vi "Main_ch.vi"() -> ()   [LabVIEW 2020]
uses:
  <vilib>/Utility/error.llb/DialogType.ctl
  <vilib>/DAQmx/read.llb/DAQmx Read (Analog 1D Wfm NChan NSamp).vi
  <extravilib>/ChannelInstances/Tag-bool/Read With Abort.vi
  <extravilib>/ChannelInstances/Tag-bool/Write With Abort.vi
  <vilib>/ULx/Create Channel.llb/ULx Create Channel (AI-Voltage-Basic).vi
  <vilib>/ULx/Timing.llb/ULx Timing (Sample Clock).vi
  <vilib>/DAQmx/create/channels.llb/DAQmx Create Channel (AI-Acceleration-Accelerometer).vi
  <vilib>/DAQmx/configure/timing.llb/DAQmx Timing (Sample Clock).vi
  <vilib>/DAQmx/configure/trigger.llb/DAQmx Start Trigger (Digital Edge).vi
  <vilib>/DAQmx/configure/trigger.llb/DAQmx Start Trigger (Time).vi
  <vilib>/DAQmx/configure/trigger.llb/DAQmx Start Trigger (Analog Edge).vi
  <extravilib>/ChannelInstances/Tag-bool/Instantiate.vi
  <extravilib>/ChannelInstances/Tag-bool/EndpointRead.vi
  <vilib>/ULx/Read.llb/ULx Read (Analog Wfm 1Chan NSamp).vi
  <vilib>/DAQmx/miscellaneous.llb/DAQmx Fill In Error Info.vi
  <vilib>/ULx/Read.llb/ULx Read (Analog 1D Wfm NChan NSamp).vi
  <instrlib>/Tektronix DPO MSO 2000 4000 Series/Public/Data/Read (Multiple Waveforms).vi
  <vilib>/Waveform/WDTFileIO.llb/Export Waveforms To Spreadsheet File (1D).vi
  <extravilib>/ChannelInstances/Tag-bool/Endpoint.vi
  <extravilib>/ChannelInstances/Tag-bool.lvlib
  <instrlib>/Tektronix DPO MSO 2000 4000 Series/Tektronix DPO MSO 2000 4000 Series.lvlib
  <resource>/objmgr/daqmx.rc
panel:
  out "Power Graph":waveform(dbl)[](graph)
  out "Torque Graph":waveform(dbl)(graph)
  in  "Trigger Type":T1(tab)
  in  "Digital Start Trigger Edge":i32(ring)=10280 caption="Edge" items=["Rising"=10280, "Falling"=10171]
  in  "Digital Start Trigger Source":tag="/Dev1/PFI0" caption="Source"
  in  "Digital Pause Trigger Pause When":i32(ring)=10192 caption="Pause When" items=["High"=10192, "Low"=10214]
  in  "Digital Pause Trigger Source":tag="/Dev1/PFI0" caption="Source"
  in  "Analog Start Trigger Level":dbl caption="Level" format="%0.2f"
  in  "Analog Start Trigger Hysteresis":dbl caption="Hysteresis" format="%.2f"
  in  "Analog Start Trigger Slope":i32(ring)=10280 caption="Slope" items=["Rising"=10280, "Falling"=10171]
  in  "Analog Start Trigger Source":string="APFI0" caption="Source"
  in  "Analog Pause Trigger Source":string="APFI0" caption="Source"
  in  "Analog Pause Trigger Pause When":i32(ring)=10093 caption="Pause When" items=["Above Level"=10093, "Below Level"=10107]
  in  "Analog Pause Trigger Level":dbl caption="Level" format="%.2f"
  in  "When":timestamp
  in  "Select Time\nManually":bool
  out "Waveform Graph":waveform(dbl)[](graph)
  out "Actual Sample Rate":dbl=1000.0 format="%0.2f"
  out "Mic Graph":dynamicdata(graph)
  out "Load Cell Graph":waveform(dbl)[](graph)
  in  "stop":bool
  # "To enable triggers, select a tab above, and configure the settings.\n\nNot all hardware supports all trigger types. Refer to your device documentation for more information."
  # "This trigger type is not supported in continuous sample timing. \n\nRefer to your device documentation for more information on which triggers are supported."
  # "This trigger type is not supported in continuous sample timing. \n\nRefer to your device documentation for more information on which triggers are supported."
  # "If time is not manually set, task will begin after 10 seconds"
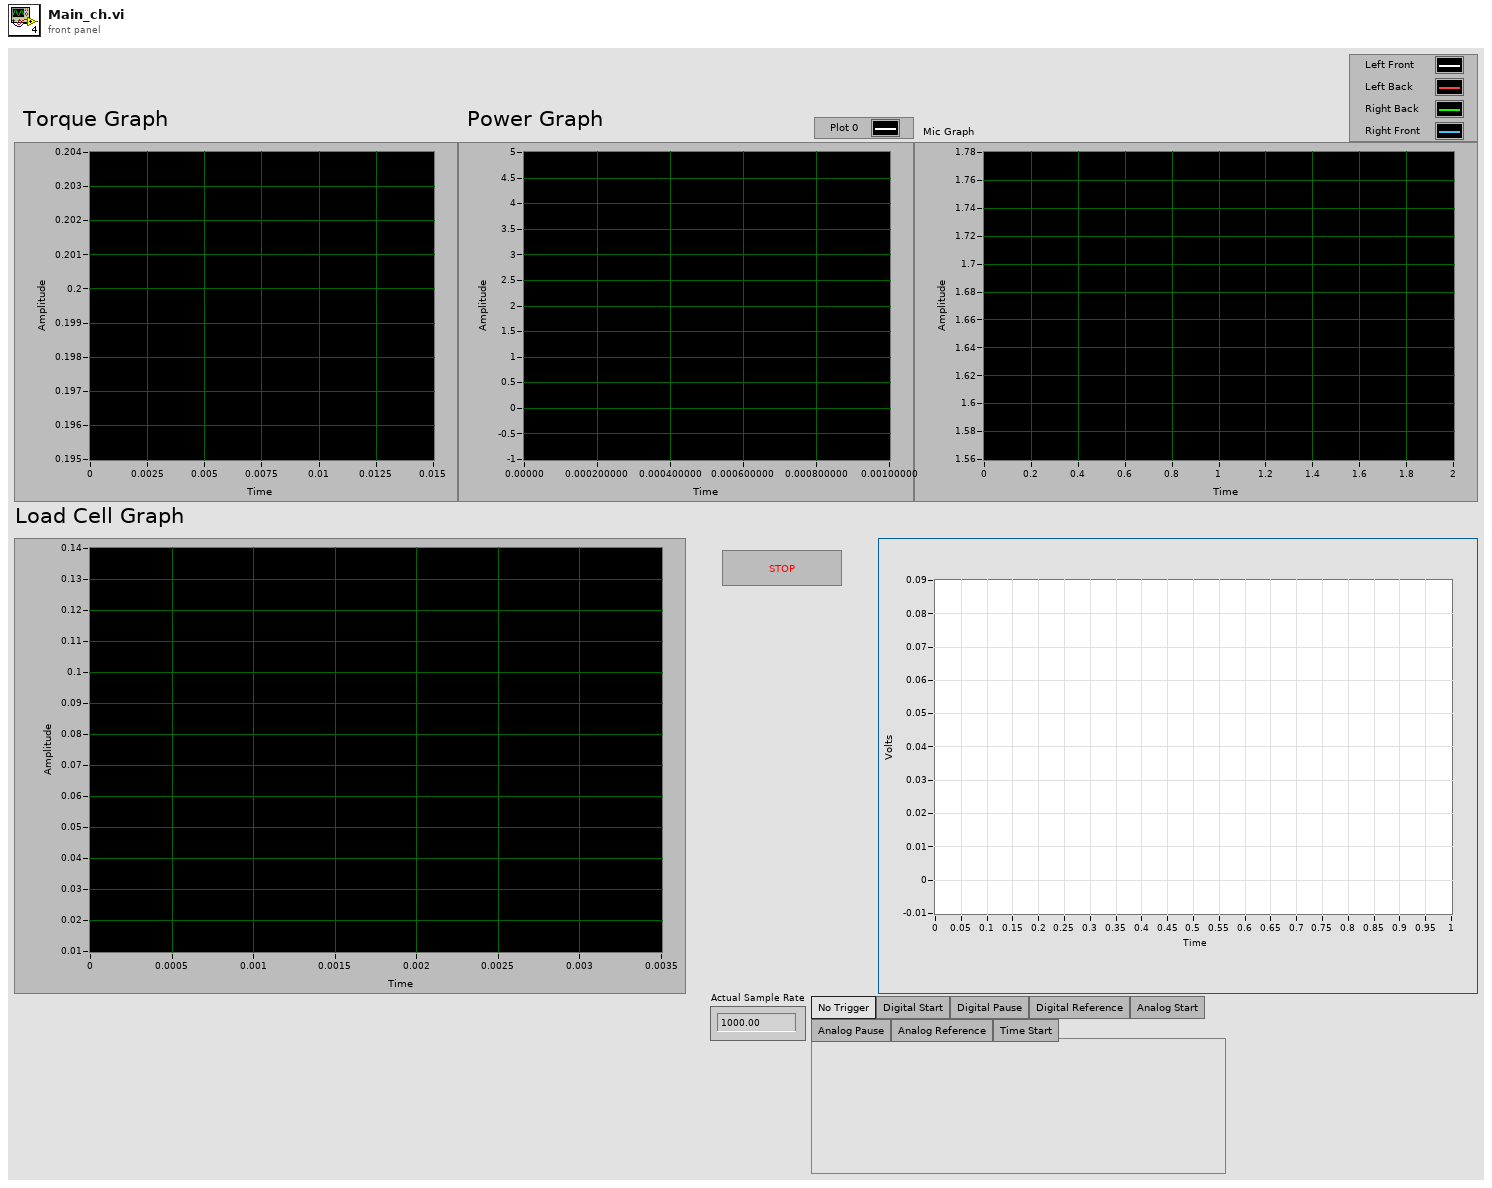
[diagram p1: front panel]
types:
  T1 = enum32{"No Trigger", "Digital Start", "Digital Pause", "Digital Reference", "Analog Start", "Analog Pause", "Analog Reference", "Time Start"}
  T2 = typedef "DialogType.ctl" = u16
  T3 = typedef "Tag-bool.lvlib/))Channel.ctl" = refnum<queue>
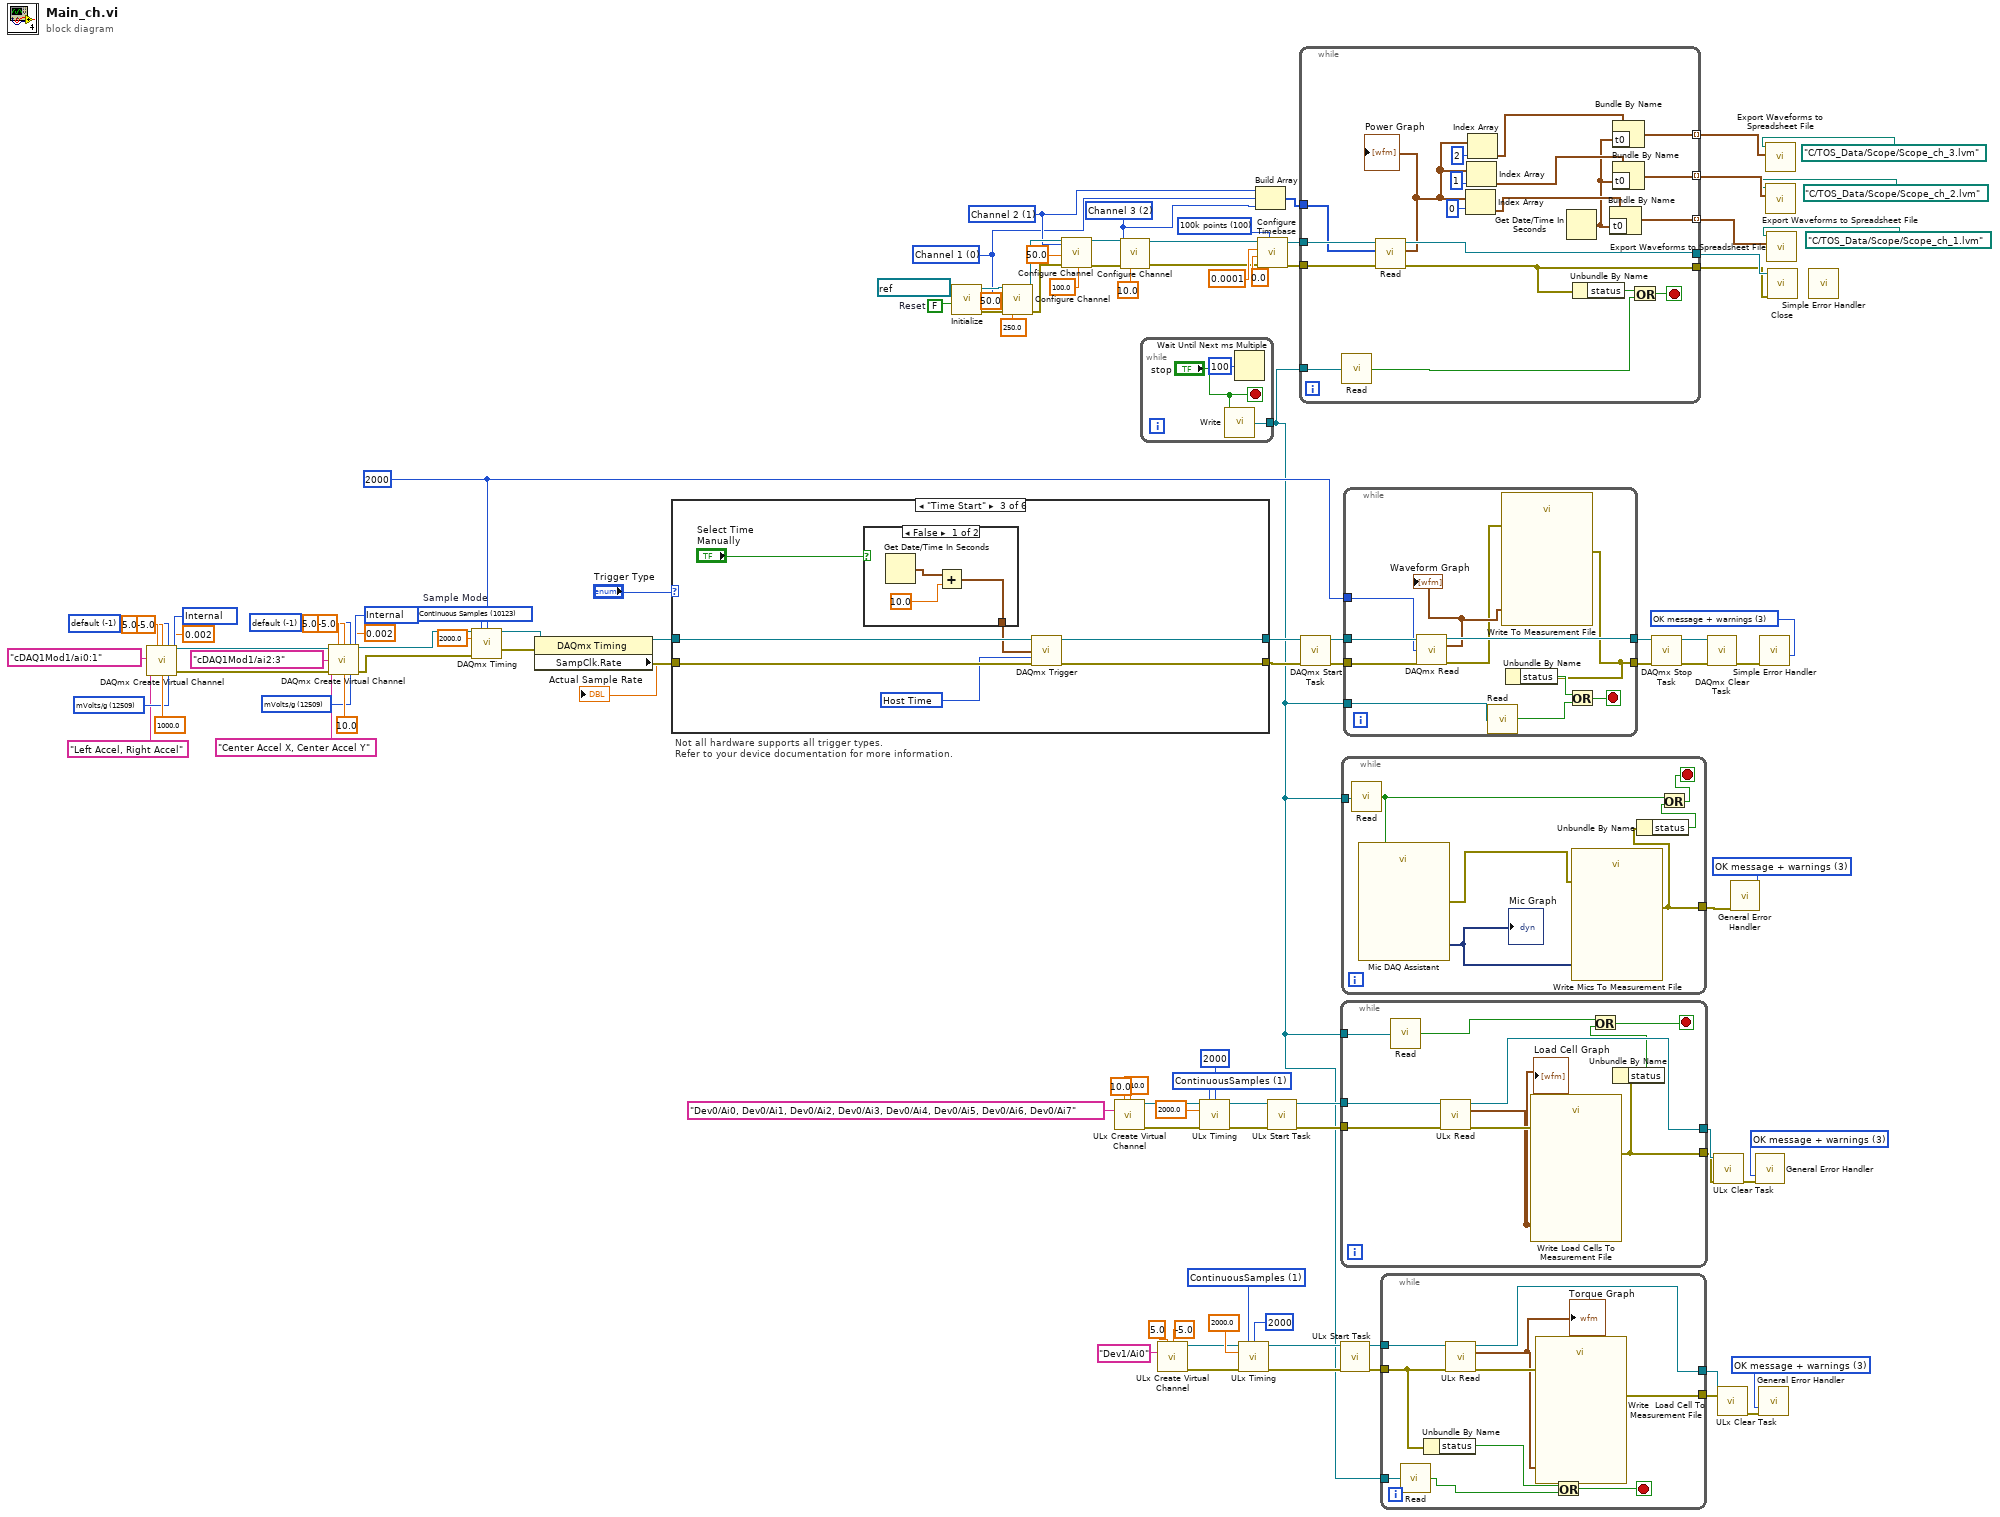
[diagram p0: block diagram]
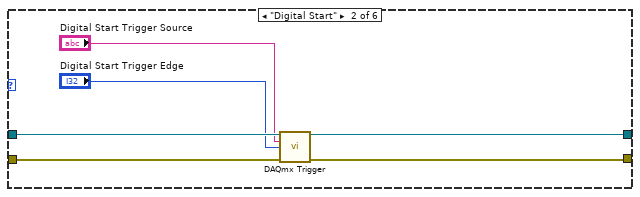
[diagram p3: hidden frame]
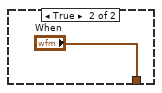
[diagram p4: hidden frame]
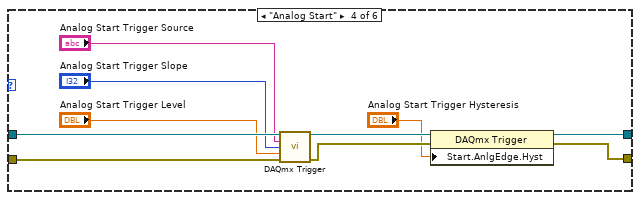
[diagram p5: hidden frame]
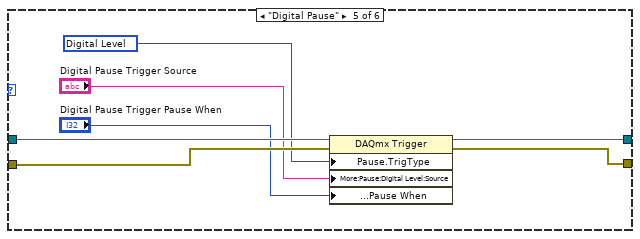
[diagram p6: hidden frame]
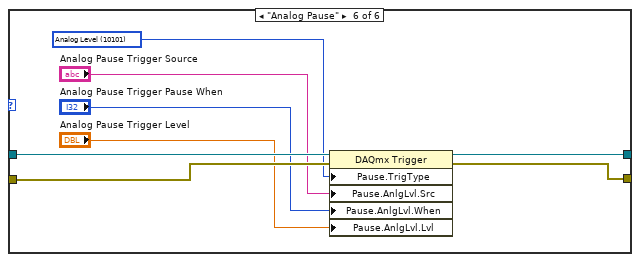
[diagram p7: hidden frame]
diagram:
  w13 = u16 2 items=["Channel 1", "Channel 2", "Channel 3", "Channel 4", "Math", "Reference 1", "Reference 2", "Reference 3", "Reference 4", "Bus 1", "Bus 2"] ("Channel (0: Channel 1)")
  w31 = 1 items=["FiniteSamples", "ContinuousSamples"] ("sample mode")
  w28 = T2 3 items=["no dialog", "OK message", "continue or stop message", "OK message + warnings", "continue/stop + warnings"] ("type of dialog (OK msg:1)")
  w46 = 12509 items=["mVolts/g"=12509, "Volts/g"=12510] ("sensitivity units")
  w47 = 12509 items=["mVolts/g"=12509, "Volts/g"=12510] ("sensitivity units")
  w51 = 10200 items=["Internal"=10200, "External"=10167, "None"=10230] ("current excitation source")
  w52 = -1 items=["default"=-1, "RSE"=10083, "NRSE"=10078, "Differential"=10106, "Pseudodifferential"=12529] ("input terminal configuration")
  w56 = 2000 ("samples per channel")
  w61 = T2 3 items=["no dialog", "OK message", "continue or stop message", "OK message + warnings", "continue/stop + warnings"] ("type of dialog (OK msg:1)")
  w72 = 10123 items=["Finite Samples"=10178, "Continuous Samples"=10123, "Hardware Timed Single Point"=12522]  # Sample Mode
  w76 = 10200 items=["Internal"=10200, "External"=10167, "None"=10230] ("current excitation source")
  w77 = -1 items=["default"=-1, "RSE"=10083, "NRSE"=10078, "Differential"=10106, "Pseudodifferential"=12529] ("input terminal configuration")
  w81 = T2 3 items=["no dialog", "OK message", "continue or stop message", "OK message + warnings", "continue/stop + warnings"] ("type of dialog (OK msg:1)")
  w41 = u16 1 items=["Channel 1", "Channel 2", "Channel 3", "Channel 4", "Math", "Reference 1", "Reference 2", "Reference 3", "Reference 4", "Bus 1", "Bus 2"] ("Channel (0: Channel 1)")
  w40 = u16 0 items=["Channel 1", "Channel 2", "Channel 3", "Channel 4", "Math", "Reference 1", "Reference 2", "Reference 3", "Reference 4", "Bus 1", "Bus 2"] ("Channel (0: Channel 1)")
  w91 = u32 100 items=["1000 points"=1, "10k points"=10, "100k points"=100, "1M points"=1000, "5M points"=5000, "10M points"=10000] ("Record Length (10: 10k points)")
  w83 = FALSE  # Reset
  w97 = 1 items=["FiniteSamples", "ContinuousSamples"] ("sample mode")
  w101 = T2 3 items=["no dialog", "OK message", "continue or stop message", "OK message + warnings", "continue/stop + warnings"] ("type of dialog (OK msg:1)")
  # "Not all hardware supports all trigger types.\nRefer to your device documentation for more information."
  n1 = call-poly <vilib>:"DAQmx Create Virtual Channel.vi"("maximum value"=5.0, "minimum value"=-5.0, "input terminal configuration"=w77, "physical channels"=tag "cDAQ1Mod1/ai0:1", "current excitation source"=w76, "name to assign"="Left Accel, Right Accel", "current excitation value"=0.002, "sensitivity"=1000.0, "sensitivity units"=w46) -> ("task out"=w43:refnum<k21>, "error out"=w44:errorcluster)  [unwired: 5 in]
  n2 = call-poly <vilib>:"DAQmx Create Virtual Channel.vi"("task in"=w43, "maximum value"=5.0, "minimum value"=-5.0, "input terminal configuration"=w52, "physical channels"=tag "cDAQ1Mod1/ai2:3", "current excitation source"=w51, "name to assign"="Center Accel X, Center Accel Y", "current excitation value"=0.002, "error in"=w44, "sensitivity"=10.0, "sensitivity units"=w47) -> ("task out"=w42:refnum<k21>, "error out"=w45:errorcluster)  [unwired: 3 in]
  n3 = call-poly <vilib>:"DAQmx Timing.vi"("task/channels in"=w42, "sample mode"=w72, "samples per channel"=w56, "rate"=2000.0, "error in"=w45) -> ("task out"=w74:refnum<k21>, "error out"=w73:errorcluster)  [unwired: 9 in]
  n4 = property class="DAQmx Timing"(reference=w74, error in=w73) -> (reference out=w71:refnum<k21>, error out=w70:errorcluster, "SampClk.Rate"=→"Actual Sample Rate":dbl)
  n5 = case shown="\"Time Start\"" "Trigger Type" {
    tunnel: w71 -> [w110 w116 w123 w137 w144 w152]
    tunnel: w70 -> [w109 w115 w122 w136 w141 w149]
    tunnel: [w110 w114 w121 w134 w143 w151] -> w58
    tunnel: [w109 w113 w120 w133 w142 w150] -> w59
    frame "No Trigger", Default {
    }
    frame "Digital Start" {
      n6 = call-poly <vilib>:"DAQmx Trigger.vi"("task/channels in"=w116, "source"="Digital Start Trigger Source", "edge"="Digital Start Trigger Edge", "error in"=w115) -> ("task out"=w114:refnum<k21>, "error out"=w113:errorcluster)  [unwired: 10 in]
    }
    frame "Time Start" {
      w119 = 16126 items=["Host Time"=16126, "I/O Device Time"=16127] ("timescale")
      n7 = case shown="False" "Select Time\nManually" {
        tunnel: [w124 "When"] -> w117
        frame False {
          n8 = Get Date/Time In Seconds() -> (seconds since 1Jan1904=w126:timestamp)
          n9 = Add(x=w126, y=10.0) -> (x+y=w124:timestamp)
        }
        frame True {
        }
      }
      n10 = call-poly <vilib>:"DAQmx Trigger.vi"("task/channels in"=w123, "when"=w117, "timescale"=w119, "error in"=w122) -> ("task out"=w121:refnum<k21>, "error out"=w120:errorcluster)  [unwired: 10 in]
    }
    frame "Analog Start" {
      n11 = call-poly <vilib>:"DAQmx Trigger.vi"("task/channels in"=w137, "source"="Analog Start Trigger Source", "slope"="Analog Start Trigger Slope", "level"="Analog Start Trigger Level", "error in"=w136) -> ("task out"=w132:refnum<k21>, "error out"=w131:errorcluster)  [unwired: 9 in]
      n12 = property class="DAQmx Trigger"(reference=w132, error in=w131, "Start.AnlgEdge.Hyst"="Analog Start Trigger Hysteresis") -> (reference out=w134:refnum<k21>, error out=w133:errorcluster)
    }
    frame "Digital Pause" {
      w140 = 10152 items=["Analog Level"=10101, "Analog Window"=10103, "Digital Level"=10152, "Digital Pattern"=10398, "None"=10230] ("Pause.TrigType")
      n13 = property class="DAQmx Trigger"(reference=w144, error in=w141, "Pause.TrigType"=w140, "More:Pause:Digital Level:Source"="Digital Pause Trigger Source", "More:Pause:Digital Level:Pause When"="Digital Pause Trigger Pause When") -> (reference out=w143:refnum<k21>, error out=w142:errorcluster)
    }
    frame "Analog Pause" {
      w148 = 10101 items=["Analog Level"=10101, "Analog Window"=10103, "Digital Level"=10152, "Digital Pattern"=10398, "None"=10230] ("Pause.TrigType")
      n14 = property class="DAQmx Trigger"(reference=w152, error in=w149, "Pause.TrigType"=w148, "Pause.AnlgLvl.Src"="Analog Pause Trigger Source", "Pause.AnlgLvl.When"="Analog Pause Trigger Pause When", "Pause.AnlgLvl.Lvl"="Analog Pause Trigger Level") -> (reference out=w151:refnum<k21>, error out=w150:errorcluster)
    }
  }
  n15 = call <instrlib>:"Initialize.vi"("Reset (True)"=w83, "VISA resource name"=refnum<visa-resource-name> "MSO3014") -> ("error out"=w89:errorcluster, "VISA resource name out"=w90:refnum<visa-resource-name>)  [unwired: 8 in]
  n16 = call <instrlib>:"Configure Channel.vi"("VISA resource name"=w90, "Channel (0: Channel 1)"=w40, "Probe Attenuation (1)"=50.0, "error in (no error)"=w89, "Vertical Range (10.0 V)"=250.0) -> ("VISA resource name out"=w88:refnum<visa-resource-name>, "error out"=w87:errorcluster)  [unwired: 9 in]
  n17 = call <instrlib>:"Configure Channel.vi"("VISA resource name"=w88, "Channel (0: Channel 1)"=w41, "Probe Attenuation (1)"=50.0, "error in (no error)"=w87, "Vertical Range (10.0 V)"=100.0) -> ("VISA resource name out"=w18:refnum<visa-resource-name>, "error out"=w15:errorcluster)  [unwired: 9 in]
  n18 = call-poly <vilib>:"ULx Create Virtual Channel.vi"("maximum value"=10.0, "minimum value"=-10.0, "physical channels"="Dev0/Ai0, Dev0/Ai1, Dev0/Ai2, Dev0/Ai3, Dev0/Ai4, Dev0/Ai5, Dev0/Ai6, Dev0/Ai7") -> ("task out"=w105:refnum<k24>, "error out"=w108:errorcluster)  [unwired: 11 in]
  n19 = call <instrlib>:"Configure Channel.vi"("VISA resource name"=w18, "Channel (0: Channel 1)"=w13, "error in (no error)"=w15, "Vertical Range (10.0 V)"=10.0) -> ("VISA resource name out"=w17:refnum<visa-resource-name>, "error out"=w16:errorcluster)  [unwired: 10 in]
  n20 = while {
    tunnel: [w153] -> w1
    stop <- "stop" stop-if-true
    n21 = call <extravilib>:"Write.vi"("element"="stop") -> ("channel"=w153:T3)  [unwired: 1 out]
    n22 = Wait Until Next ms Multiple(millisecond multiple=u32 100 ("millisecond timer value")) -> ()  [unwired: 1 out]
  }
  n23 = call-poly <vilib>:"ULx Create Virtual Channel.vi"("maximum value"=5.0, "minimum value"=-5.0, "physical channels"="Dev1/Ai0") -> ("task out"=w24:refnum<k24>, "error out"=w21:errorcluster)  [unwired: 11 in]
  n24 = call-poly <vilib>:"ULx Timing.vi"("task in"=w105, "sample mode"=w97, "samples per channel"=2000, "rate"=2000.0, "error in"=w108) -> ("task out"=w38:refnum<k24>, "error out"=w100:errorcluster)  [unwired: 9 in]
  n25 = call-poly <vilib>:"ULx Timing.vi"("task in"=w24, "sample mode"=w31, "samples per channel"=2000, "rate"=2000.0, "error in"=w21) -> ("task out"=w29:refnum<k24>, "error out"=w30:errorcluster)  [unwired: 9 in]
  n26 = Build Array(w41, w40, w13) -> (w4:u16[])
  n27 = call <instrlib>:"Configure Timebase.vi"("Record Length (10: 10k points)"=w91, "error in (no error)"=w16, "Position (10 %)"=0.0, "Timebase (0.0005 s)"=0.0001, "VISA resource name"=w17) -> ("error out"=w2:errorcluster, "VISA resource name out"=w3:refnum<visa-resource-name>)  [unwired: 5 in]
  n28 = call <vilib>:"ULx Start Task.vi"("task in"=w38, "error in"=w100) -> ("task out"=w104:refnum<k24>, "error out"=w107:errorcluster)  [unwired: 12 in]
  n29 = while {
    tunnel: w3 -> [w175]
    tunnel: w2 -> [w174]
    tunnel: [w173] -> w12
    tunnel: w4 -> [w171]
    tunnel: [w169] -> w11
    tunnel: [w166] -> w10 mode=indexing
    tunnel: [w159] -> w9 mode=indexing
    tunnel: [w158] -> w8 mode=indexing
    tunnel: w1 -> [w157]
    stop <- w170 stop-if-true
    n30 = call <instrlib>:"Read.vi"("channel"=w157) -> ("element"=w156:bool)  [unwired: 1 in, 1 out]
    n31 = call-poly <instrlib>:"Read.vi"("error in (no error)"=w174, "Channels"=w171, "VISA resource name"=w175) -> ("error out"=w169:errorcluster, "Waveform Data"=w163:waveform(dbl)[], "VISA resource name out"=w173:refnum<visa-resource-name>)  [unwired: 6 in]
    "Power Graph" <- w163
    n32 = Index Array(array=w163, index=0) -> (element=w167:waveform(dbl))
    n33 = Index Array(array=w163, index=1) -> (element=w161:waveform(dbl))
    n34 = Index Array(array=w163, index=2) -> (element=w162:waveform(dbl))
    n35 = Get Date/Time In Seconds() -> (seconds since 1Jan1904=w160:timestamp)
    n36 = Unbundle By Name(w169) -> ("status"=w172:bool)
    n37 = Bundle By Name(cluster=w167, "t0"=w160) -> (w166:waveform(dbl))
    n38 = Bundle By Name(cluster=w162, "t0"=w160) -> (w158:waveform(dbl))
    n39 = Bundle By Name(cluster=w161, "t0"=w160) -> (w159:waveform(dbl))
    n40 = Or(x=w172, y=w156) -> (x .or. y?=w170:bool)
  }
  n41 = call <vilib>:"DAQmx Start Task.vi"("task/channels in"=w58, "error in"=w59) -> ("task out"=w69:refnum<k21>, "error out"=w68:errorcluster)  [unwired: 12 in]
  n42 = while {
    tunnel: w107 -> [w181]
    tunnel: w104 -> [w185]
    tunnel: [w184] -> w103
    tunnel: [w176] -> w102
    tunnel: w1 -> [w179]
    stop <- w183 stop-if-true
    n43 = call <instrlib>:"Read.vi"("channel"=w179) -> ("element"=w177:bool)  [unwired: 1 in, 1 out]
    n44 = call-poly <vilib>:"ULx Read.vi"("task in"=w185, "error in"=w181) -> ("task out"=w184:refnum<k24>, "data"=w180:waveform(dbl)[], "error out"=w182:errorcluster)  [unwired: 11 in]
    "Load Cell Graph" <- w180
    n45 = call "Write Load Cells To Measurement File"("Signals"=w180, "error in (no error)"=w182) -> ("error out"=w176:errorcluster)  [unwired: 15 in, 2 out]
    n46 = Unbundle By Name(w176) -> ("status"=w178:bool)
    n47 = Or(x=w177, y=w178) -> (x .or. y?=w183:bool)
  }
  n48 = call <vilib>:"ULx Start Task.vi"("task in"=w29, "error in"=w30) -> ("task out"=w25:refnum<k24>, "error out"=w22:errorcluster)  [unwired: 12 in]
  n49 = while {
    tunnel: w1 -> [w191]
    tunnel: [w186] -> w82
    stop <- w189 stop-if-true
    n50 = call <instrlib>:"Read.vi"("channel"=w191) -> ("element"=w187:bool)  [unwired: 1 in, 1 out]
    n51 = call "Mic DAQ Assistant"("stop (T)"=w187) -> ("data"=w192:dynamicdata, "error out"=w190:errorcluster)  [unwired: 16 in, 1 out]
    "Mic Graph" <- w192
    n52 = call "Write Mics To Measurement File"("Signals"=w192, "error in (no error)"=w190) -> ("error out"=w186:errorcluster)  [unwired: 15 in, 2 out]
    n53 = Unbundle By Name(w186) -> ("status"=w188:bool)
    n54 = Or(x=w187, y=w188) -> (x .or. y?=w189:bool)
  }
  n55 = while {
    tunnel: w69 -> [w203]
    tunnel: w68 -> [w202]
    tunnel: [w201] -> w65
    tunnel: [w193] -> w64
    tunnel: w56 -> [w198]
    tunnel: w1 -> [w196]
    stop <- w199 stop-if-true
    n56 = call-poly <vilib>:"DAQmx Read.vi"("task/channels in"=w203, "number of samples per channel"=w198, "error in"=w202) -> ("task out"=w201:refnum<k21>, "data"=w195:waveform(dbl)[], "error out"=w194:errorcluster)  [unwired: 10 in]
    "Waveform Graph" <- w195
    n57 = call <instrlib>:"Read.vi"("channel"=w196) -> ("element"=w197:bool)  [unwired: 1 in, 1 out]
    n58 = call "Write To Measurement File"("Signals"=w195, "error in (no error)"=w194) -> ("error out"=w193:errorcluster)  [unwired: 15 in, 2 out]
    n59 = Unbundle By Name(w193) -> ("status"=w200:bool)
    n60 = Or(x=w200, y=w197) -> (x .or. y?=w199:bool)
  }
  n61 = while {
    tunnel: w22 -> [w207]
    tunnel: w25 -> [w213]
    tunnel: [w212] -> w26
    tunnel: [w208] -> w27
    tunnel: w1 -> [w206]
    stop <- w210 stop-if-true
    n62 = call <instrlib>:"Read.vi"("channel"=w206) -> ("element"=w205:bool)  [unwired: 1 in, 1 out]
    n63 = Unbundle By Name(w207) -> ("status"=w211:bool)
    n64 = call-poly <vilib>:"ULx Read.vi"("task in"=w213, "error in"=w207) -> ("task out"=w212:refnum<k24>, "data"=w204:waveform(dbl), "error out"=w209:errorcluster)  [unwired: 11 in]
    "Torque Graph" <- w204
    n65 = call "Write  Load Cell To Measurement File"("Signals"=w204, "error in (no error)"=w209) -> ("error out"=w208:errorcluster)  [unwired: 15 in, 2 out]
    n66 = Or(x=w211, y=w205) -> (x .or. y?=w210:bool)
  }
  n67 = call <vilib>:"DAQmx Stop Task.vi"("task/channels in"=w65, "error in"=w64) -> ("task out"=w62:refnum<k21>, "error out"=w63:errorcluster)  [unwired: 12 in]
  n68 = call <vilib>:"DAQmx Clear Task.vi"("task in"=w62, "error in"=w63) -> ("error out"=w67:errorcluster)  [unwired: 13 in]
  n69 = call <vilib>:"ULx Clear Task.vi"("task in"=w103, "error in"=w102) -> ("error out"=w106:errorcluster)  [unwired: 13 in]
  n70 = call <vilib>:"ULx Clear Task.vi"("task in"=w26, "error in"=w27) -> ("error out"=w23:errorcluster)  [unwired: 13 in]
  n71 = call <vilib>:"General Error Handler.vi"("type of dialog (OK msg:1)"=w81, "error in (no error)"=w82) -> ()  [unwired: 9 in, 5 out]
  n72 = call <vilib>:"General Error Handler.vi"("type of dialog (OK msg:1)"=w101, "error in (no error)"=w106) -> ()  [unwired: 9 in, 5 out]
  n73 = call <vilib>:"General Error Handler.vi"("type of dialog (OK msg:1)"=w28, "error in (no error)"=w23) -> ()  [unwired: 9 in, 5 out]
  n74 = call <vilib>:"Simple Error Handler.vi"("type of dialog (OK msg:1)"=w61, "error in (no error)"=w67) -> ()  [unwired: 3 in, 5 out]
  n75 = call-poly <vilib>:"Export Waveforms to Spreadsheet File.vi"("waveforms"=w8, "file path (dialog if empty)"=path "C:/TOS_Data/Scope/Scope_ch_3.lvm") -> ()  [unwired: 8 in, 2 out]
  n76 = call-poly <vilib>:"Export Waveforms to Spreadsheet File.vi"("waveforms"=w9, "file path (dialog if empty)"=path "C:/TOS_Data/Scope/Scope_ch_2.lvm") -> ()  [unwired: 8 in, 2 out]
  n77 = call-poly <vilib>:"Export Waveforms to Spreadsheet File.vi"("waveforms"=w10, "file path (dialog if empty)"=path "C:/TOS_Data/Scope/Scope_ch_1.lvm") -> ()  [unwired: 8 in, 2 out]
  n78 = call <instrlib>:"Close.vi"("error in (no error)"=w11, "VISA resource name"=w12) -> ()  [unwired: 9 in, 1 out]
  n79 = call <vilib>:"Simple Error Handler.vi"() -> ()  [unwired: 5 in, 5 out]
